vi "Write Single Pin Height to File.vi"(6 "Error at file writing":errorcluster, 7 "File Path for saving measurements":path, 8 "Image Name":string="20170125_164904.835_IMGA.png", 9 "Pin Height (microns)":dbl, 10 "Pin Height (Pixels)":dbl, 11 "Pin Number":dbl) -> (0 "Error out at file writing":errorcluster, 3 "File Path of saved file":path)   [LabVIEW 2016]
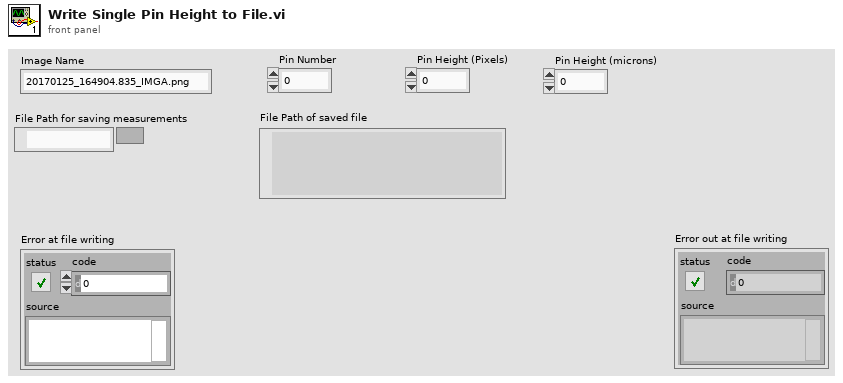
[diagram p1: front panel]
types:
  T1 = enum16{"open", "replace", "create", "open or create", "replace or create", "replace or create with confirmation"}
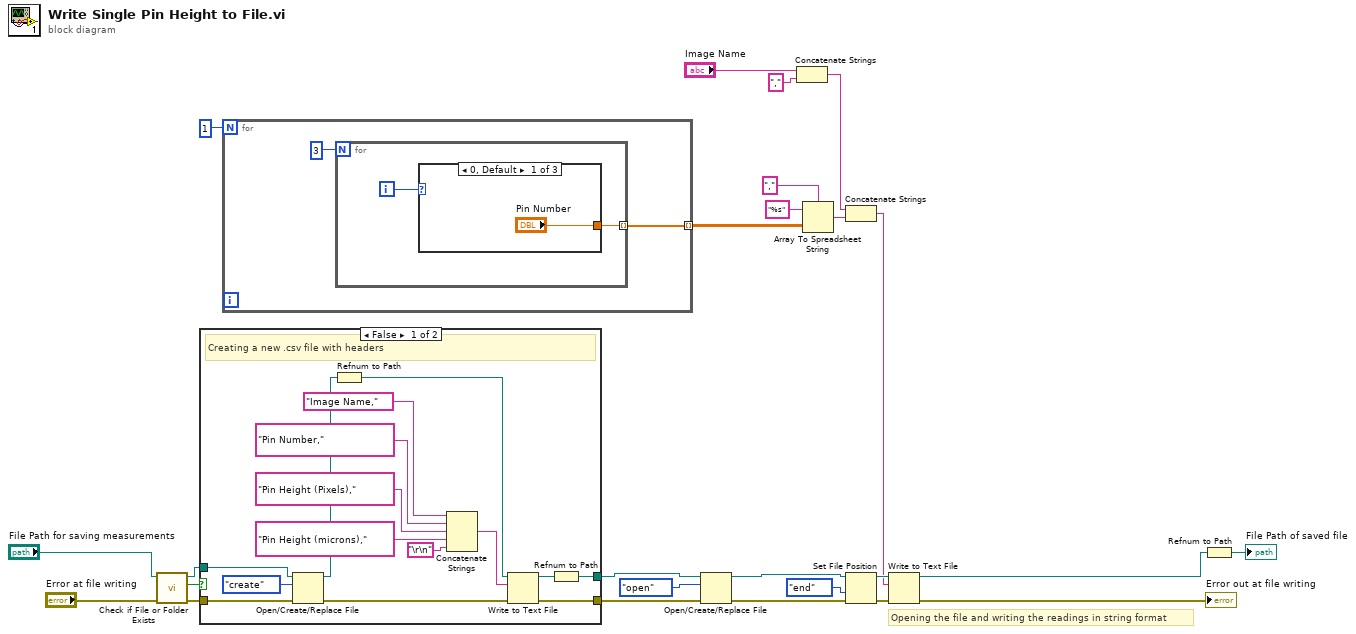
[diagram p0: block diagram]
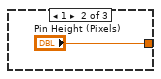
[diagram p3: hidden frame]
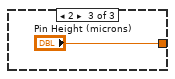
[diagram p4: hidden frame]
diagram:
  # "Opening the file and writing the readings in string format"
  n1 = call <vilib>:"Check if File or Folder Exists.vi"("error in (no error)"="Error at file writing", "path"="File Path for saving measurements") -> ("error out"=w4:errorcluster, "file or folder exists?"=w5:bool, "dup path"=w2:path)  [unwired: 7 in]
  n2 = case shown="False" w5 {
    tunnel: [w31 w42] -> w3
    tunnel: w4 -> [w38 w42]
    tunnel: w2 -> [w40 w41]
    tunnel: [w33 w41] -> w1
    frame False {
      # "Creating a new .csv file with headers"
      n3 = Open/Create/Replace File(file path (use dialog)=w40, error in=w38, operation (0:open)=T1."create") -> (refnum out=w37:refnum<file>, error out=w32:errorcluster)  [unwired: 3 in, 1 out]
      n4 = Refnum to Path(1:w37) -> (0:w35:path)
      n5 = Concatenate Strings("Image Name," ("string"), "Pin Number," ("string"), "Pin Height (Pixels)," ("string"), "Pin Height (microns)," ("string"), "\r\n") -> (w36:string)
      n6 = Write to Text File(file (use dialog)=w35, text=w36, error in=w32) -> (refnum out=w34:refnum<file>, error out=w31:errorcluster)  [unwired: 1 in, 1 out]
      n7 = Refnum to Path(1:w34) -> (0:w33:path)
    }
    frame True {
      # "If the file exists then the data is wriiten to .csv file"
    }
  }
  n8 = for {
    N: 1 -> [_]
    tunnel: [w43] -> w8 mode=indexing
    n9 = for {
      N: 3 ("Numeric") -> [_]
      tunnel: [w45] -> w43 mode=indexing
      i -> [w46]
      n10 = case shown="0, Default" w46 {
        tunnel: ["Pin Number" "Pin Height (Pixels)" "Pin Height (microns)"] -> w45
        frame 0, Default {
        }
        frame 1 {
        }
        frame 2 {
        }
      }
    }
  }
  n11 = Open/Create/Replace File(file path (use dialog)=w1, error in=w3, operation (0:open)=T1."open") -> (refnum out=w21:refnum<file>, error out=w12:errorcluster)  [unwired: 3 in, 1 out]
  n12 = Concatenate Strings("Image Name", "," ("delimiter (\\t)")) -> (w17:string)
  n13 = Array To Spreadsheet String(delimiter (Tab)="," ("delimiter (\\t)"), array=w8, 3:"%s" ("format string")) -> (spreadsheet string=w15:string)
  n14 = Concatenate Strings(w17, w15) -> (w20:string)
  n15 = Set File Position(refnum=w21, from (0:start)=enum16{"start", "end", "current"}."end", error in=w12) -> (refnum out=w23:refnum<file>, error out=w19:errorcluster)  [unwired: 1 in]
  n16 = Write to Text File(file (use dialog)=w23, text=w20, error in=w19) -> (refnum out=w10:refnum<file>, error out=→"Error out at file writing":errorcluster)  [unwired: 1 in, 1 out]
  n17 = Refnum to Path(1:w10) -> (0:→"File Path of saved file":path)
